vi "Line Clock Control.vi"(9 "line clock in":i32, 10 "Elements per line":i32, 11 "output valid? in":bool) -> (3 "line clock out":i32)   [LabVIEW 2015]
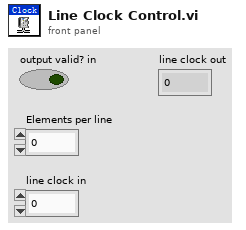
[diagram p1: front panel]
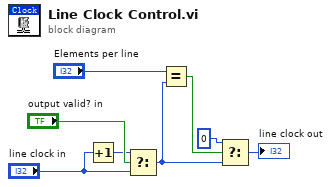
[diagram p0: block diagram]
diagram:
  n1 = Increment(x="line clock in") -> (x+1=w2:i32)
  n2 = Select(t=w2, s="output valid? in", f="line clock in") -> (s? t:f=w4:i32)
  n3 = Equal?(x="Elements per line", y=w4) -> (x = y?=w3:bool)
  n4 = Select(t=0, s=w3, f=w4) -> (s? t:f=→"line clock out":i32)
